vi "hysteresis_PI.vi"(7 "N_hyst":i32, 8 "y_vec_in":sgl[](array[numeric])=[0.0, 0.0, 0.0, 0.0, 0.0, 0.0, 0.0], 9 "w_s":sgl[](array[numeric])=[0.0, 0.0, 0.0, 0.0, 0.0, 0.0, 0.0], 10 "r_s":sgl[](array[numeric])=[0.0, 0.0, 0.0, 0.0, 0.0, 0.0, 0.0], 11 "uk":sgl format="%#_13g") -> (0 "y_vec_out":sgl[](array[numeric]), 3 "H_of_ik":sgl)   [LabVIEW 2017]
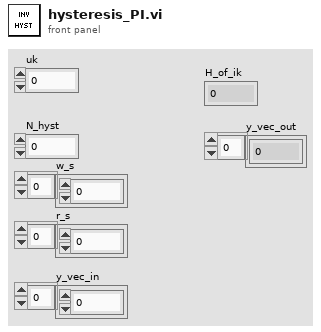
[diagram p1: front panel]
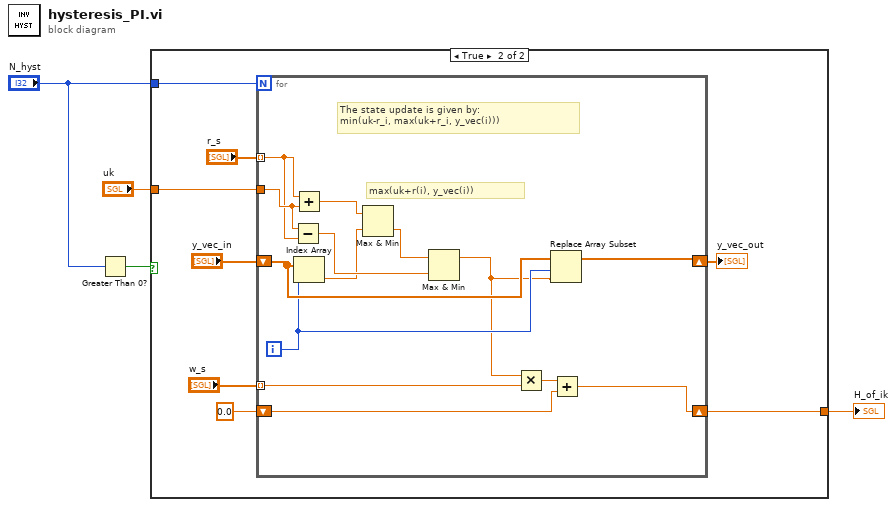
[diagram p0: block diagram]
diagram:
  n1 = Greater Than 0?(x="N_hyst") -> (x > 0?=w2:bool)
  n2 = case shown="True" w2 {
    tunnel: "N_hyst" -> [_ w13]
    tunnel: [w5 w7] -> w4
    tunnel: "uk" -> [w5 w6]
    frame False {
    }
    frame True {
      n3 = for {
        N: w13 -> [_]
        tunnel: "w_s" -> [w21] mode=indexing
        tunnel: "r_s" -> [w25] mode=indexing
        shift-right: [w18] -> w7
        shift-left: sgl 0.0 -> [w19]
        tunnel: w6 -> [w26]
        shift-right: [w17] -> w8
        shift-left: "y_vec_in" -> [w16]
        i -> [w15]
        # "max(uk+r(i), y_vec(i))"
        # "The state update is given by:\nmin(uk-r_i, max(uk+r_i, y_vec(i)))"
        n4 = Subtract(x=w26, y=w25) -> (x-y=w23:sgl)
        n5 = Add(x=w25, y=w26) -> (x+y=w27:sgl)
        n6 = Index Array(array=w16, index=w15) -> (element=w22:sgl)
        n7 = Max & Min(x=w27, y=w22) -> (min(x,y)=w24:sgl)  [unwired: 1 out]
        n8 = Max & Min(x=w24, y=w23) -> (max(x,y)=w14:sgl)  [unwired: 1 out]
        n9 = Multiply(x=w14, y=w21) -> (x*y=w20:sgl)
        n10 = Replace Array Subset(array=w16, new element=w14, index=w15) -> (w17:sgl[])
        n11 = Add(x=w20, y=w19) -> (x+y=w18:sgl)
      }
      "y_vec_out" <- w8
    }
  }
  "H_of_ik" <- w4
